vi "DestroyModuleEvents.vi"(8 "error in (no error)":errorcluster, 11 "JQMHModule in":refnum<class "RQMHModule.lvclass">) -> (0 "error out":errorcluster, 3 "JQMHModule out":refnum<class "RQMHModule.lvclass">)   [LabVIEW 2024, in "RQMHModule.lvclass"]
uses:
  RQMHModule.lvclass
  RQMHModule.lvclass/RQMHModule.ctl
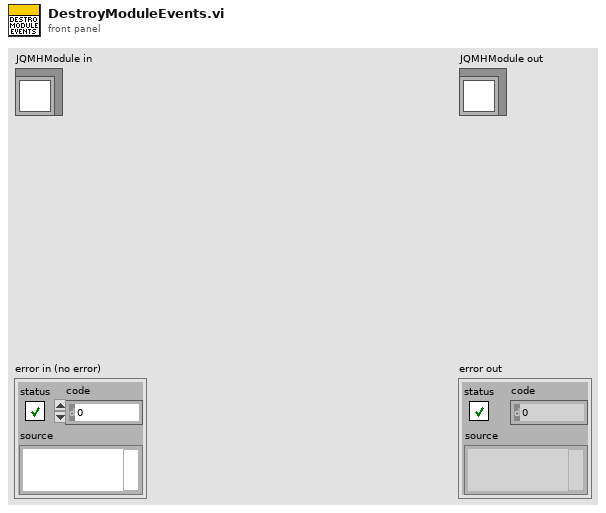
[diagram p1: front panel]
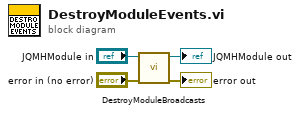
[diagram p0: block diagram]
diagram:
  n1 = call-dynamic "DestroyModuleBroadcasts.vi"("error in (no error)"="error in (no error)", "JQMHModule in"="JQMHModule in") -> ("error out"=→"error out":errorcluster, "JQMHModule out"=→"JQMHModule out":refnum<class "RQMHModule.lvclass">)  [unwired: 8 in]
